vi "Start Log and Sequence.vi"(5 "WorkspaceManager":T2, 6 "Log File Path":path, 7 "Test Columns in":T4, 8 "error in (no error)":errorcluster, 9 "Log Config Name (CSVDataLog)":string="CSVDataLog", 10 "Log Trigger Name (CSVSeqLogTrigger)":string="CSVSeqLogTrigger", 11 "Stim Session":T3) -> (0 "error out":errorcluster, 1 "Session Complete Event Ref":T1, 2 "WorkspaceManager out":T2, 3 "Stim Session out":T3)   [LabVIEW 2011]
uses:
  Controls/CSVs Tests Data.ctl
  Controls/Test Column Data.ctl
  <vilib>/NI Veristand/Execution/Workspace/WorkspaceAPI.ctl
  NationalInstruments.VeriStand.ClientAPI
  <vilib>/NI Veristand/Execution/SequenceExecutionInterface/Stimulus Profile Session Ref.ctl
  <vilib>/NI Veristand/Execution/SequenceExecutionInterface/Session Event Ref.ctl
  <vilib>/NI Veristand/Execution/Workspace/LogFileConfiguration.ctl
  <vilib>/NI Veristand/Execution/Workspace/LogFileTriggerConfiguration.ctl
  <vilib>/NI Veristand/Execution/Workspace/LogFileTriggerType.ctl
  <vilib>/NI Veristand/Execution/Workspace/LogProperty.ctl
  <vilib>/NI Veristand/Execution/Workspace/LogChannelConfiguration.ctl
  <vilib>/NI Veristand/Execution/Workspace/NI VeriStand - Get Alias List.vi
  <vilib>/NI Veristand/Execution/Workspace/NI VeriStand - Get System Node Channel List.vi
  <vilib>/NI Veristand/Execution/Workspace/NI_VS Workspace ExecutionAPI.lvlib
  <vilib>/NI Veristand/Execution/SequenceExecutionInterface/NI_VS Sequence Execution Interface.lvlib
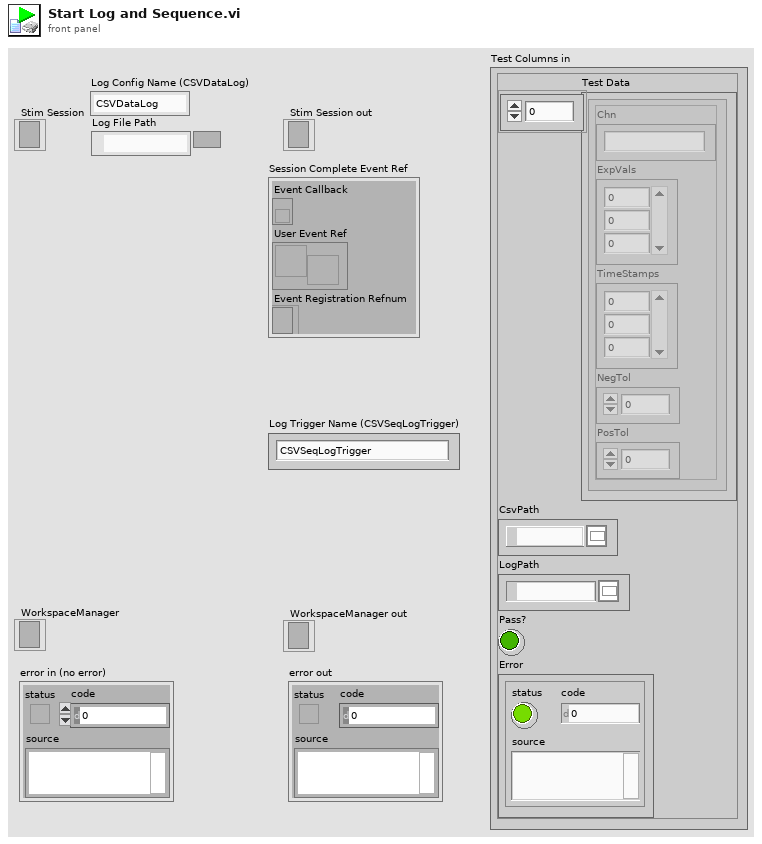
[diagram p1: front panel]
types:
  T1 = typedef "NI_VS Sequence Execution Interface.lvlib/Session Event Ref.ctl" = cluster{"Event Callback":refnum<k27>, "User Event Ref":refnum<user-event>, "Event Registration Refnum":refnum<event-registration>}
  T2 = typedef "NI_VS Workspace ExecutionAPI.lvlib/WorkspaceAPI.ctl" = refnum<k24>
  T3 = typedef "NI_VS Sequence Execution Interface.lvlib/Stimulus Profile Session Ref.ctl" = refnum<k24>
  T4 = typedef "CSVs Tests Data.ctl" = cluster{"Test Data":T5[], "CsvPath":path, "LogPath":path, "Pass?":bool, "Error":errorcluster}
  T5 = typedef "Test Column Data.ctl" = cluster{"Chn":string, "ExpVals":dbl[], "TimeStamps":i64[], "NegTol":dbl, "PosTol":dbl}
  T6 = typedef "NI_VS Workspace ExecutionAPI.lvlib/LogChannelConfiguration.ctl" = cluster{"Channel Path":string, "Custom Name":string, "Custom Group":string, "Properties":T7[]}
  T7 = typedef "NI_VS Workspace ExecutionAPI.lvlib/LogProperty.ctl" = cluster{"Name":string, "Value":string}
  T8 = typedef "NI_VS Workspace ExecutionAPI.lvlib/LogFileTriggerType.ctl" = enum16{"None", "In Limits", "Out of Limits"}
  T9 = typedef "NI_VS Workspace ExecutionAPI.lvlib/LogFileTriggerConfiguration.ctl" = cluster{"Type":T8, "Channel Path":string, "High Limit":dbl, "Low Limit":dbl}
  T10 = typedef "NI_VS Workspace ExecutionAPI.lvlib/LogFileConfiguration.ctl" = cluster{"File Path":path, "Description":string, "Trigger":T9, "Replace File":bool, "Rate [Hz]":dbl, "File Properties":T7[], "Channels":T6[]}
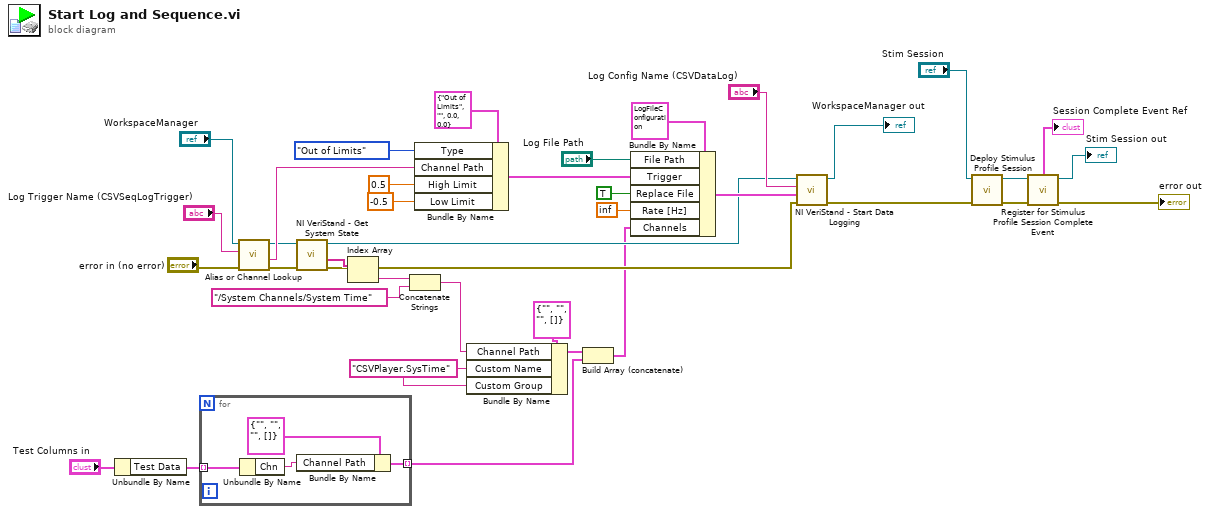
[diagram p0: block diagram]
diagram:
  w3 = "CSVPlayer.SysTime" ("Custom Name")
  n1 = Unbundle By Name("Test Columns in") -> ("Test Data"=w1:T5[])
  n2 = for {
    tunnel: w1 -> [w42] mode=indexing
    tunnel: [w39] -> w6 mode=indexing
    n3 = Unbundle By Name(w42) -> ("Chn"=w40:string)
    n4 = Bundle By Name(cluster=T6 {"Channel Path"="", "Custom Name"="", "Custom Group"="", "Properties"=[]} ("LogChannelInfo"), "Channel Path"=w40) -> (w39:T6)
  }
  n5 = call "Alias or Channel Lookup.vi"("error in (no error)"="error in (no error)", "Item"="Log Trigger Name (CSVSeqLogTrigger)", "WorkspaceManager in"="WorkspaceManager") -> ("error out"=w15:errorcluster, "Channel"=w16:string, "WorkspaceManager out"=w14:T2)  [unwired: 5 in, 1 out]
  n6 = call <vilib>:"NI VeriStand - Get System State.vi"("error in (no error)"=w15, "WorkspaceManager in"=w14) -> ("error out"=w12:errorcluster, "Targets"=w13:string[], "WorkspaceManager  out"=w11:T2)  [unwired: 5 in, 2 out]
  n7 = Index Array(array=w13) -> (element=w10:string)  [unwired: 1 in]
  n8 = Concatenate Strings(w10, "/System Channels/System Time" ("string")) -> (w4:string)
  n9 = Bundle By Name(cluster=T9 {"Type"=enum."Out of Limits", "Channel Path"="", "High Limit"=0.0, "Low Limit"=0.0} ("Trigger"), "Type"=LogFileTriggerType."Out of Limits", "Channel Path"=w16, "High Limit"=0.5, "Low Limit"=-0.5) -> (w29:T9)
  n10 = Bundle By Name(cluster=T6 {"Channel Path"="", "Custom Name"="", "Custom Group"="", "Properties"=[]} ("LogChannelInfo"), "Channel Path"=w4, "Custom Name"=w3, "Custom Group"=w3) -> (w7:T6)
  n11 = Build Array (concatenate)(w7, w6) -> (w5:T6[])
  n12 = Bundle By Name(cluster=T10 {"File Path"=path "", "Description"="", "Trigger"={"Type"=enum."None", "Channel Path"="", "High Limit"=0.0, "Low Limit"=0.0}, "Replace File"=FALSE, "Rate [Hz]"=1.0, "File Properties"=[], "Channels"=[]} ("Data Log File Configuration"), "File Path"="Log File Path", "Trigger"=w29, "Replace File"=TRUE, "Rate [Hz]"=inf, "Channels"=w5) -> (w25:T10)
  n13 = call <vilib>:"NI VeriStand - Start Data Logging.vi"("error in (no error)"=w12, "Data Log File Configuration"=w25, "Data Log Configuration Name"="Log Config Name (CSVDataLog)", "WorkspaceManager in"=w11) -> ("error out"=w2:errorcluster, "WorkspaceManager out"=→"WorkspaceManager out":T2)  [unwired: 6 in]
  n14 = call <vilib>:"Deploy Stimulus Profile Session.vi"("error in (no error)"=w2, "Session Ref in"="Stim Session") -> ("error out"=w24:errorcluster, "Session Ref out"=w23:T3)  [unwired: 7 in, 1 out]
  n15 = call <vilib>:"Register for Stimulus Profile Session Complete Event.vi"("error in (no error)"=w24, "Session Ref in"=w23) -> ("error out"=→"error out":errorcluster, "Session Ref out"=→"Stim Session out":T3, "Session Complete Event Ref"=→"Session Complete Event Ref":T1)  [unwired: 6 in, 1 out]
